vi "RT Main.vi"() -> ()   [LabVIEW 2017]
uses:
  <vilib>/myRIO/Instrument Drivers/Onboard IO/I2C/typedefs/I2C User Configuration.ctl
  <vilib>/myRIO/Instrument Drivers/Onboard IO/I2C/typedefs/I2C Transfer Rate.ctl
  <vilib>/Platform/TimedLoop/XDataNode/timing_clust.ctl
  <vilib>/Platform/TimedLoop/XDataNode/nitl_modes.ctl
  <vilib>/Platform/TimedLoop/XDataNode/wakeup.ctl
  <vilib>/myRIO/Instrument Drivers/Onboard IO/I2C/typedefs/I2C Reference.ctl
  <vilib>/myRIO/Common/Instrument Driver Framework/Utilities/typedefs/myRIO Generic Hardware Reference.ctl
  <vilib>/myRIO/Common/Instrument Driver Framework/Utilities/typedefs/Hardware Version Enum.ctl
  <vilib>/myRIO/Common/Instrument Driver Framework/Utilities/typedefs/myRIO v1.0 Reference.ctl
  <vilib>/myRIO/Common/Instrument Driver Framework/Utilities/typedefs/Generic FPGA Reference.ctl
  <vilib>/myRIO/Common/Instrument Driver Framework/myRIO v1.0/I2C/typedefs/I2C Channels Enum.ctl
  <vilib>/myRIO/Instrument Drivers/Onboard IO/I2C/typedefs/I2C Configuration.ctl
  <vilib>/userdefined/High Color/nirio_resource_hc.ctl
  <vilib>/myRIO/Common/Instrument Driver Framework/Utilities/vis/Is FPGA Ref Available.vi
  <vilib>/myRIO/Common/Instrument Driver Framework/myRIO v1.0/I2C/vis/myRIO v1.1 Open I2C.vi
  <vilib>/myRIO/Common/Instrument Driver Framework/Utilities/vis/Validate Channels.vi
  <vilib>/myRIO/Common/Instrument Driver Framework/myRIO v1.0/I2C/vis/myRIO v1.0 Reserve I2C.vi
  <vilib>/Analysis/baseanly.llb/Outer Product.vi
  <vilib>/Analysis/baseanly.llb/Real Outer Product.vi
  <vilib>/robotics/Kinematics/Create Lie Group Matrix.vi
  <vilib>/myRIO/Common/Instrument Driver Framework/myRIO v1.0/UART/vis/myRIO v1.0 Close UART.vi
  <vilib>/myRIO/Common/Instrument Driver Framework/myRIO v1.0/I2C/vis/myRIO v1.0 Build MUX Configuration I2C.vi
  <vilib>/myRIO/Common/Instrument Driver Framework/myRIO v1.0/Resource Manager/vis/myRIO v1.0 Reserve Channel List.vi
  <vilib>/myRIO/Common/Instrument Driver Framework/myRIO v1.0/Resource Manager/vis/myRIO v1.0 Create Configuration List.vi
  <vilib>/myRIO/Common/Instrument Driver Framework/myRIO v1.0/Resource Manager/vis/myRIO v1.0 Reserve Channel.vi
  <vilib>/myRIO/Common/Instrument Driver Framework/myRIO v1.0/Resource Manager/vis/myRIO v1.0 Unreserve Channel.vi
  <vilib>/myRIO/Common/Instrument Driver Framework/myRIO v1.0/Resource Manager/vis/myRIO v1.0 Build Mutex Name.vi
  <vilib>/Utility/error.llb/Error Cluster From Error Code.vi
  <vilib>/myRIO/Common/Instrument Driver Framework/myRIO v1.0/I2C/vis/myRIO v1.0 Configure I2C.vi
  <vilib>/myRIO/Common/Instrument Driver Framework/myRIO v1.0/I2C/vis/myRIO v1.0 Write I2C.vi
  <vilib>/myRIO/Common/Instrument Driver Framework/myRIO v1.0/I2C/vis/myRIO v1.0 Read I2C.vi
  <vilib>/Utility/VariantDataType/GetNumericInfo.vi
  <vilib>/myRIO/Common/Instrument Driver Framework/myRIO v1.0/myRIO v1.1 Open.vi
  <vilib>/myRIO/Common/Instrument Driver Framework/Utilities/vis/IO Manager.vi
  <vilib>/myRIO/Common/Instrument Driver Framework/Utilities/vis/Configuration Manager.vi
  <vilib>/myRIO/Common/Instrument Driver Framework/myRIO v1.0/Resource Manager/vis/myRIO v1.0 Configure IO.vi
  <vilib>/myRIO/Common/Instrument Driver Framework/myRIO v1.0/myRIO v1.0 Close.vi
  <vilib>/Analysis/Matrix/Numeric/Multiply/Multiply.vi
  <vilib>/Analysis/Matrix/Numeric/Multiply/Multiply - RM,R.vi
  <vilib>/Analysis/Matrix/Numeric/Multiply/Multiply - R,RM.vi
  <vilib>/Analysis/Matrix/Numeric/Add/Add.vi
  <vilib>/Analysis/Matrix/Numeric/Add/Add - RM,RM.vi
  <vilib>/myRIO/Common/Instrument Driver Framework/Utilities/vis/FPGA Ref Manager.vi
  <vilib>/myRIO/Common/Instrument Driver Framework/myRIO v1.0/myRIO v1.0 Reset FPGA.vi
  <vilib>/myRIO/Common/Instrument Driver Framework/myRIO v1.0/IRQ/vis/myRIO v1.0 IRQ Info FGV.vi
  <vilib>/myRIO/Common/Instrument Driver Framework/myRIO v1.0/IRQ/vis/myRIO v1.0 Timer IRQ Info FGV.vi
  <vilib>/myRIO/Common/Instrument Driver Framework/myRIO v1.0/IRQ/vis/myRIO v1.0 ISR Agent.vi
  <vilib>/platform/TimedLoop/XDataNode/XDataNode.xnode
  <vilib>/myRIO/Express VI/Onboard IO/I2C/I2C Express VI.xnode
  <vilib>/myRIO/Instrument Drivers/Onboard IO/I2C/vis/myRIO I2C Open.xnode
  <vilib>/myRIO/Instrument Drivers/Onboard IO/I2C/I2C.lvlib
  <vilib>/robotics/Kinematics/NI_Kinematics.lvlib
  <vilib>/Platform/TimedLoop/XDataNode/XDNodeRunTimeDep.lvlib
  <vilib>/myRIO/Instrument Drivers/Utilities/Utilities.lvlib
panel:
  out "Waveform Chart":dbl(graph)
  in  "stop":bool
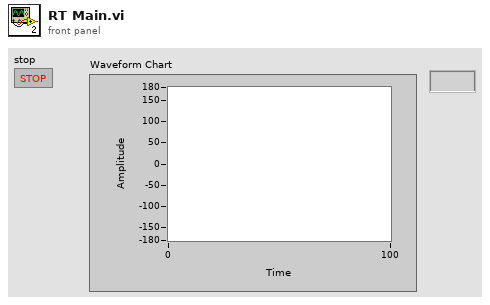
[diagram p1: front panel]
types:
  T1 = typedef "I2C.lvlib/I2C Reference.ctl" = cluster{"myRIO Reference":T2, "I2C Channels Enum":T6, "I2C Configuration":T7}
  T2 = typedef "myRIO Generic Hardware Reference.ctl" = cluster{"myRIO Model":T3, "myRIO Hardware Reference":T4}
  T3 = typedef "Hardware Version Enum.ctl" = enum16{"Unknown", "myRIO-1900", "myRIO-1950", "roboRIO", "NI ELVIS RIO CM"}
  T4 = typedef "myRIO v1.0 Reference.ctl" = cluster{"Generic FPGA Reference":T5, "Allow multiple opens":bool}
  T5 = typedef "Generic FPGA Reference.ctl" = refnum<k20>
  T6 = typedef "I2C Channels Enum.ctl" = enum16{"Not Connected", "A/I2C", "B/I2C", "I2C/I2C"}
  T7 = typedef "I2C.lvlib/I2C Configuration.ctl" = cluster{"I2C Transfer Rate":T8}
  T8 = typedef "I2C.lvlib/I2C Transfer Rate.ctl" = enum16{"Standard mode (100 kbps)", "Fast mode (400 kbps)"}
  T9 = typedef "I2C.lvlib/I2C User Configuration.ctl" = cluster{"I2C Transfer Rate":T8}
  T10 = typedef "nirio_resource_hc.ctl" = tag
  T11 = typedef "XDNodeRunTimeDep.lvlib/timing_clust.ctl" = cluster{"Expected End [f-1]":u64, "Actual End [f-1]":u64, "Finished Late? [f-1]":bool, "Expected End [i-1]":u64, "Actual End [i-1]":u64, "Finished Late? [i-1]":bool, "Expected Start [i]":u64, "Actual Start [i]":u64, "Expected Start [f]":u64, "Actual Start [f]":u64, "Source Name":string, "Structure Name":string, "Period":i64, "Deadline":i64, "Offset":i64, "Start":i64, "Priority":i32, "Timeout":i32, "Mode":T12, "Wakeup Reason":T13, "Error":errorcluster, "Source Type":string, "Secondary Source Type":string, "Global End Time":u64, "Global Start Time":u64, "Frame Duration":u64, "Iteration Duration":u64, "Assigned CPU":i32, "I/O Scan Engine Mode":u32}
  T12 = typedef "XDNodeRunTimeDep.lvlib/nitl_modes.ctl" = enum32{"No Change", "Process missed periods, maintain original phase", "Discard missed periods, maintain original phase", "Process missed periods, ignore original phase", "Discard missed periods, ignore original phase"}
  T13 = typedef "XDNodeRunTimeDep.lvlib/wakeup.ctl" = enum32{"Normal", "Aborted", "Asynchronous wakeup", "Timing source error", "Timed loop error", "Timeout"}
  T14 = typedef "NI_Matrix.lvlib/RealMatrix.ctl" = dbl[][]
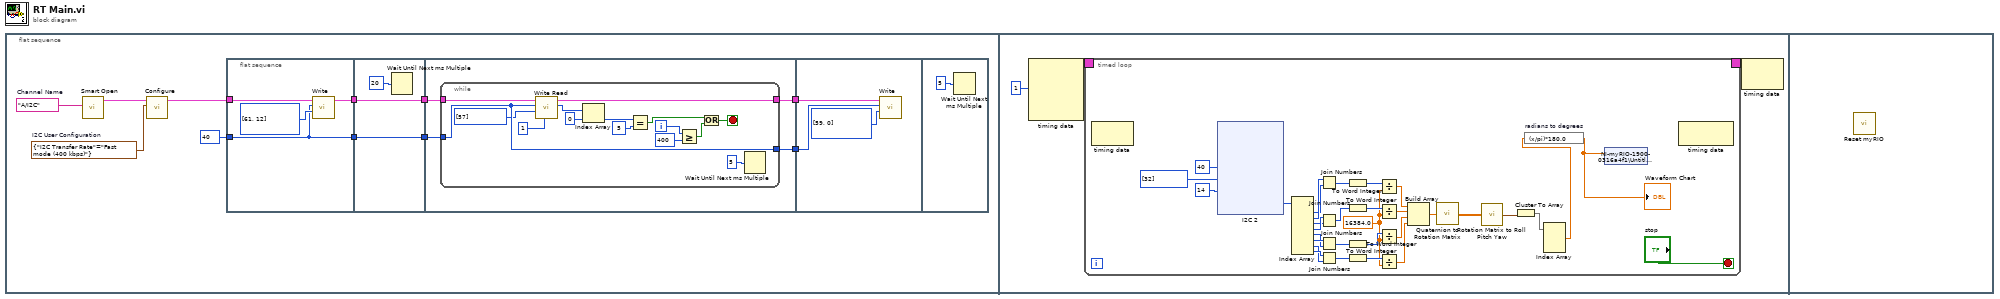
[diagram p0: block diagram]
diagram:
  n1 = flat-sequence {
    frame #0 {
      w2 = tag "A/I2C"  # Channel Name
      w1 = T9 {"I2C Transfer Rate"=enum."Fast mode (400 kbps)"}  # I2C User Configuration
      n2 = call <vilib>:"Smart Open.vi"("Channel Name"=w2) -> ("I2C Ref Out"=w3:T1)  [unwired: 9 in, 1 out]
      n3 = call <vilib>:"Configure.vi"("I2C User Configuration"=w1, "I2C Ref In"=w3) -> ("I2C Ref Out"=w4:T1)  [unwired: 8 in, 1 out]
      n4 = flat-sequence {
        tunnel: w4 -> [w14]
        tunnel: u8 40 ("Slave Address (7-bit)") -> [w12]
        tunnel: [w13] -> w11
        tunnel: [w12] -> w10
        tunnel: [w17] -> w9
        tunnel: w11 -> [w17]
        tunnel: w10 -> [w16]
        tunnel: [w16] -> w8
        tunnel: w9 -> [w22]
        tunnel: w8 -> [w21]
        tunnel: [w20] -> w7
        tunnel: [w19] -> w6
        tunnel: w7 -> [w38]
        tunnel: w6 -> [w39]
        frame #0 {
          n5 = call <vilib>:"Write.vi"("Bytes to Write"=u8[] [61, 12], "Slave Address (7-bit)"=w12, "I2C Ref In"=w14) -> ("I2C Ref Out"=w13:T1)  [unwired: 7 in, 1 out]
        }
        frame #1 {
          n6 = Wait Until Next ms Multiple(millisecond multiple=u32 20 ("milliseconds to wait")) -> ()  [unwired: 1 out]
        }
        frame #2 {
          n7 = while {
            tunnel: w22 -> [w37]
            tunnel: w21 -> [w26]
            tunnel: [w26] -> w20
            tunnel: [w25] -> w19
            i -> [w35]
            stop <- w27 stop-if-true
            n8 = call <vilib>:"Write Read.vi"("Byte Count"=u32 1, "Bytes to Write"=u8[] [57], "Slave Address (7-bit)"=w26, "I2C Ref In"=w37) -> ("Bytes Read"=w32:u8[], "I2C Ref Out"=w25:T1)  [unwired: 4 in, 1 out]
            n9 = Index Array(array=w32, index=0) -> (element=w30:u8)
            n10 = Equal?(x=w30, y=u8 5 ("I2CBytesToRead")) -> (x = y?=w29:bool)
            n11 = Greater Or Equal?(x=w35, y=400) -> (x >= y?=w28:bool)
            n12 = Or(x=w29, y=w28) -> (x .or. y?=w27:bool)
            n13 = Wait Until Next ms Multiple(millisecond multiple=u32 5) -> ()  [unwired: 1 out]
          }
        }
        frame #3 {
          n14 = call <vilib>:"Write.vi"("Bytes to Write"=u8[] [59, 0], "Slave Address (7-bit)"=w38, "I2C Ref In"=w39) -> ()  [unwired: 7 in, 2 out]
        }
        frame #4 {
          n15 = Wait Until Next ms Multiple(millisecond multiple=u32 5) -> ()  [unwired: 1 out]
        }
      }
    }
    frame #1 {
      n16 = node-c288(i64 1 ("Period")) -> (w44:T11)  [unwired: 3 in]
      n17 = timed-loop {
        timing: w44 -> [_]
        timing-out: [_] -> w43
        stop <- "stop" stop-if-true
        w55 = 16384.0
        n18 = node-c288() -> ()  [unwired: 1 in, 1 out]
        n19 = xnode "I2C 2"("Slave Address (7-bit)"=u8 40, "Bytes to Write"=u8[] [32], "Byte Count"=u32 14) -> ("Bytes Read"=w64:u8[])  [unwired: 1 in, 1 out]
        n20 = Index Array(array=w64) -> (element #1=w65:u8, element #2=w66:u8, element #3=w67:u8, element #4=w68:u8, element #5=w69:u8, element #6=w70:u8, element #7=w71:u8, element #8=w72:u8)  [unwired: 8 in]
        n21 = Join Numbers(hi=w66, lo=w65) -> ((hi.lo)=w62:u16)
        n22 = Join Numbers(hi=w68, lo=w67) -> ((hi.lo)=w60:u16)
        n23 = Join Numbers(hi=w70, lo=w69) -> ((hi.lo)=w63:u16)
        n24 = Join Numbers(hi=w72, lo=w71) -> ((hi.lo)=w57:u16)
        n25 = To Word Integer(number=w62) -> (16bit integer=w61:i16)
        n26 = To Word Integer(number=w60) -> (16bit integer=w59:i16)
        n27 = To Word Integer(number=w63) -> (16bit integer=w58:i16)
        n28 = To Word Integer(number=w57) -> (16bit integer=w56:i16)
        n29 = Divide(x=w61, y=w55) -> (x/y=w74:dbl)
        n30 = Divide(x=w59, y=w55) -> (x/y=w75:dbl)
        n31 = Divide(x=w58, y=w55) -> (x/y=w76:dbl)
        n32 = Divide(x=w56, y=w55) -> (x/y=w51:dbl)
        n33 = Build Array(w74, w75, w76, w51) -> (w73:dbl[])
        n34 = call <vilib>:"Quaternion to Rotation Matrix.vi"("quaternion"=w73) -> ("rotation matrix"=w48:T14)
        n35 = call <vilib>:"Rotation Matrix to Roll Pitch Yaw.vi"("rotation matrix"=w48) -> ("angles"=w47:cluster{"roll":dbl, "pitch":dbl, "yaw":dbl})
        n36 = Cluster To Array(cluster=w47) -> (array=w46:dbl[])
        n37 = Index Array(array=w46) -> (element #1=w45:dbl)  [unwired: 3 in, 2 out]
        n38 = expression code="(x/pi)*180.0" "radians to degrees"(w45) -> (w49:dbl)
        "Waveform Chart" <- w49
        n39 = shared-variable "NI-myRIO-1900-0316a4f1\\Untitled Library 1.lvlib\\roll"(w49) -> ()  [unwired: 1 in, 1 out]
        n40 = node-c288() -> ()  [unwired: 1 in, 1 out]
      }
      n41 = node-c288(w43) -> ()  [unwired: 1 out]
    }
    frame #2 {
      n42 = call <vilib>:"Reset myRIO.vi"() -> ()  [unwired: 11 in, 1 out]
    }
  }
